vi "Vision Processing.vi"(4 "error in (no error)":errorcluster) -> ()   [LabVIEW 2013]
doc: "This VI runs in parallel to other tasks. It gets images from the camera, processes them for color or shape and use that information to affect robot behavior."
uses:
  <vilib>/Rock Robotics/WPI/Camera/WPI_CameraImageSize.ctl
  Robot Global Data.vi
  <vilib>/vision/NI_Vision_Development_Module.lvlib
panel:
  out "Distance, Angles out":T1(array[cluster])
  in  "Score Limits":T2={"Rect Coverage"=60.0, "X Edge Strength"=40.0, "Y Edge Strength"=60.0, "Center"=75.0, "Outer"=75.0}
  out "Original Image":T3(plugin-control)
  in  "View":bool
  in  "Area Size Limit":i32=444
  in  "Particle Count Limit":i32=10
  in  "Height of target from camera":dbl
  out "Annotated Image":T3(plugin-control)
  in  "Processing":enum32{"Color", "Intensity"}(tab)
  in  "Luminance":i32=200
  in  "Saturation":i32=50
  in  "Hue":i32(knob)=121 scale=0.0..255.0
  in  "Margins":cluster{"Hue":i32, "Sat":i32, "Lum":i32}={"Hue"=40, "Sat"=40, "Lum"=20} {"Sat" scale=0.0..40.0; "Lum" scale=0.0..40.0; "Hue" scale=0.0..40.0}
  # "This is unit-insensitive, outputs in whatever unit you feed it."
  # "Yeah, um, don't use this.\n\n[We never have, so...]"
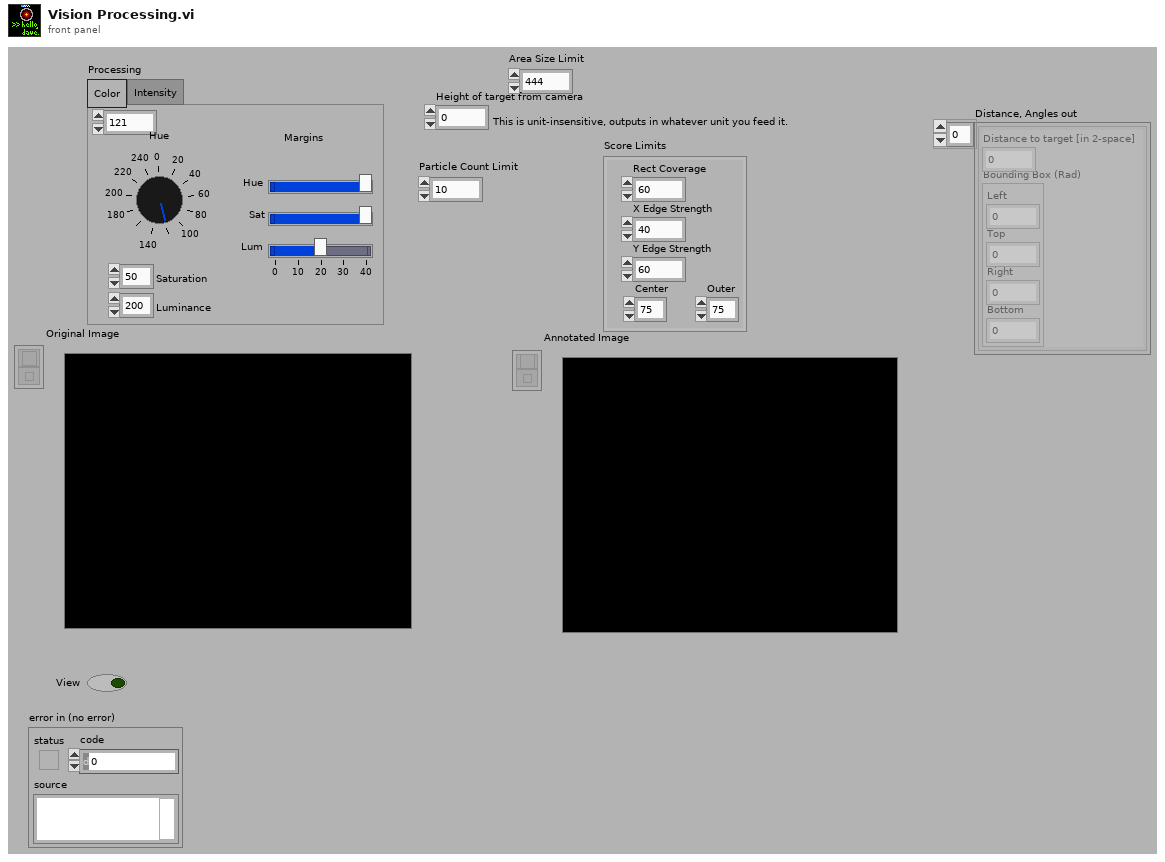
[diagram p1: front panel]
types:
  T1 = cluster{"Distance to target [in 2-space]":dbl, "Bounding Box (Rad)":cluster{"Left":dbl, "Top":dbl, "Right":dbl, "Bottom":dbl}}[]
  T2 = cluster{"Rect Coverage":dbl, "X Edge Strength":dbl, "Y Edge Strength":dbl, "Center":dbl, "Outer":dbl}
  T3 = typedef "IMAQ Image.ctl" = refnum<image>
  T4 = typedef "Image Type" = u32
  T5 = typedef "WPI_CameraDevRef.ctl" = cluster{"Camera Address":string, "CameraStatus":errorcluster, "Acquire Image Notifier":refnum<notifier>}
  T6 = typedef "CameraResolutionInfo.ctl" = cluster{"X Image Resolution":i32, "Y Image Resolution":i32, "FoV X":dbl, "FoV Y":dbl, "X scale":dbl, "Y scale":dbl}
  T7 = typedef "WPI_CameraImageSize.ctl" = enum16{"640x480", "320x240", "160x120"}
  T8 = cluster{cluster{"Left":dbl, "Top":dbl, "Right":dbl, "Bottom":dbl}, "Scores":dbl[], cluster{"Long":dbl, "Short":dbl}}[]
  T9 = cluster{"Left":dbl, "Top":dbl, "Right":dbl, "Bottom":dbl}
  T10 = cluster{"Scores[0]":dbl, "Scores[1]":dbl, "Scores[2]":dbl, "Scores[3]":dbl, "Scores[4]":dbl, "Scores[5]":dbl, "Scores[6]":dbl, "Scores[7]":dbl, "Scores[8]":dbl}
  T11 = cluster{"Distance to target [in 2-space]":dbl, "Bounding Box (Rad)":cluster{"Left":dbl, "Top":dbl, "Right":dbl, "Bottom":dbl}}
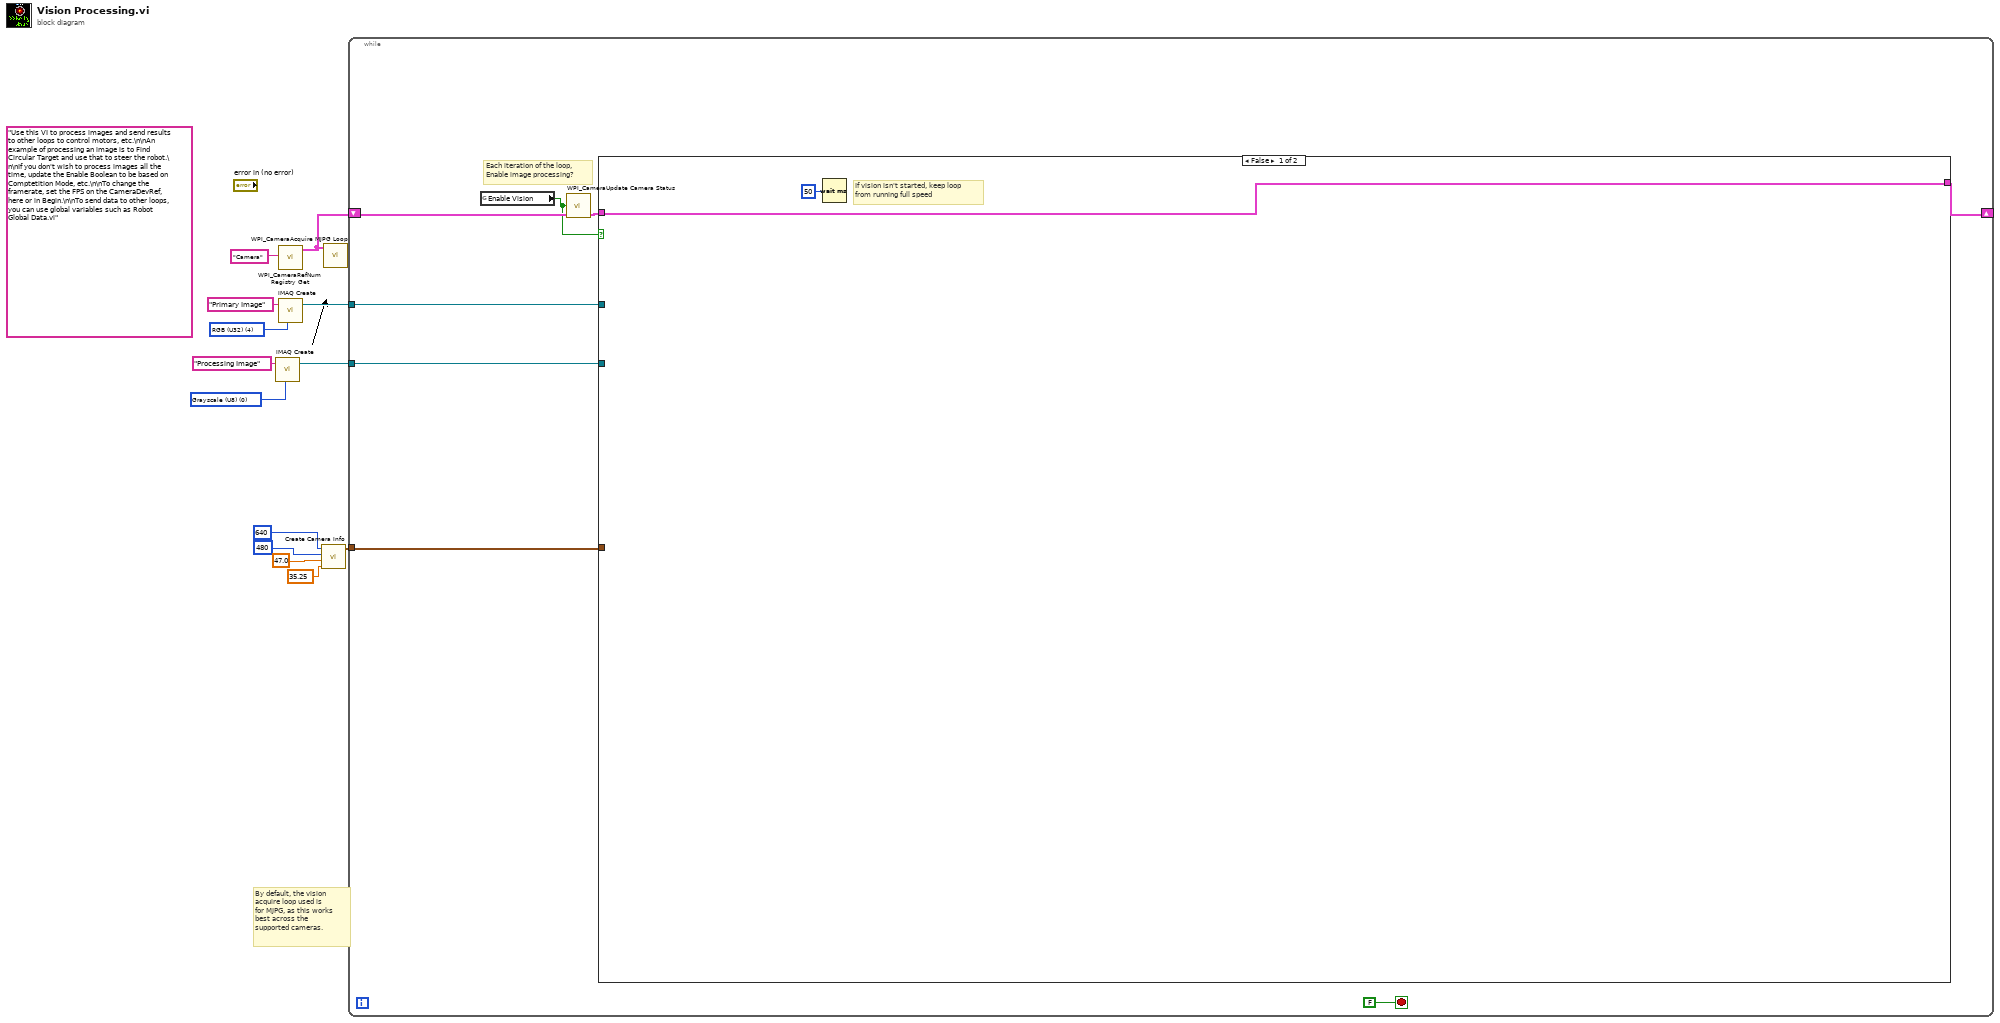
[diagram p0: block diagram]
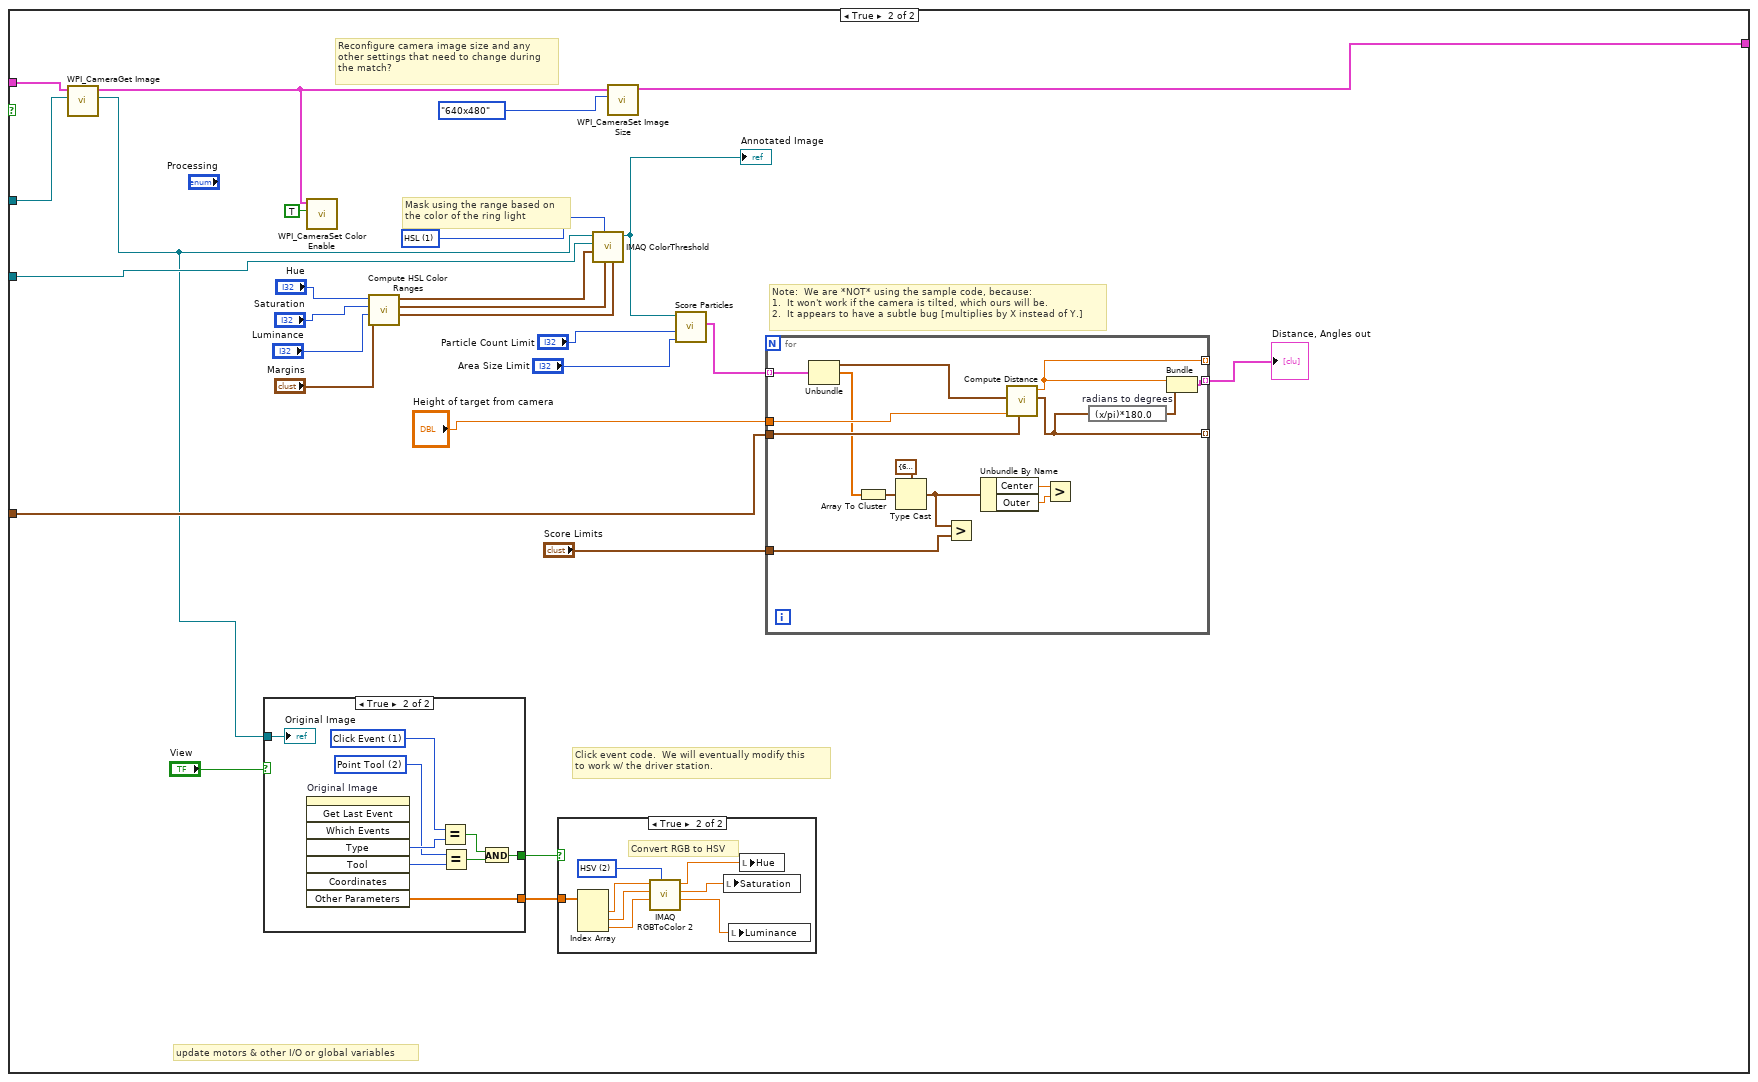
[diagram p2: hidden frame]
diagram:
  w5 = T4 0 items=["Grayscale (U8)", "Grayscale (I16)", "Grayscale (SGL)", "Complex (CSG)", "RGB (U32)", "HSL (U32)", "RGB (U64)"] ("Image Type")
  w7 = T4 4 items=["Grayscale (U8)", "Grayscale (I16)", "Grayscale (SGL)", "Complex (CSG)", "RGB (U32)", "HSL (U32)", "RGB (U64)"] ("Image Type")
  (unwired) "Use this VI to process images and send results to other loops to control motors, etc.\n\nAn example of processing an image is to Find Circular Target and use that to steer the robot.\n\nIf you don't wish to process images all the time, update the Enable Boolean to be based on Comptetition Mode, etc.\n\nTo change the framerate, set the FPS on the CameraDevRef, here or in Begin.\n\nTo send data to other loops, you can use global variables such as Robot Global Data.vi"
  # "By default, the vision\nacquire loop used is\nfor MJPG, as this works\nbest across the\nsupported cameras."
  n1 = call "IMAQ Create"("Image Name"="Processing Image", "Image Type"=w5) -> ("New Image"=w12:T3)  [unwired: 2 in, 2 out]
  n2 = call <vilib>:"WPI_CameraRefNum Registry Get.vi"("refnum name"="Camera") -> ("CameraDevRef"=w8:T5)  [unwired: 1 in, 9 out]
  n3 = call "IMAQ Create"("Image Name"="Primary Image", "Image Type"=w7) -> ("New Image"=w13:T3)  [unwired: 2 in, 2 out]
  n4 = call "Create Camera Info.vi"("FoV Y"=35.25 ("FoV X"), "FoV X"=47.0, "Y Image Resolution"=480, "X Image Resolution"=640) -> ("Camera Info"=w11:T6)  [unwired: 7 in]
  n5 = call <vilib>:"WPI_CameraAcquire MJPG Loop.vi"("CameraDevRef"=w8) -> ()  [unwired: 11 in]
  n6 = while {
    shift-right: [w20] -> _
    shift-left: w8 -> [w18]
    tunnel: w13 -> [w19]
    tunnel: w12 -> [w17]
    tunnel: w11 -> [w16]
    stop <- FALSE stop-if-true
    # "Each iteration of the loop,\nEnable image processing?"
    n7 = global read "Robot Global Data.vi" "Enable Vision"() -> (w14:bool)
    n8 = call <vilib>:"WPI_CameraUpdate Camera Status.vi"("CameraDevRef In"=w18, "Enable Vision"=w14) -> ("CameraDevRef Out"=w15:T5)  [unwired: 3 in]
    n9 = case shown="False" w14 {
      tunnel: w19 -> [_ w49]
      tunnel: [w23 w50] -> w20
      tunnel: w15 -> [w23 w48]
      tunnel: w17 -> [_ w46]
      tunnel: w16 -> [_ w45]
      frame False {
        # "If vision isn't started, keep loop\nfrom running full speed"
        n10 = Wait (ms)(milliseconds to wait=u32 50) -> ()  [unwired: 1 out]
      }
      frame True {
        w39 = u16 1 items=["RGB", "HSL", "HSV", "HSI"] ("Color Mode")
        # "Note:  We are *NOT* using the sample code, because:\n1.  It won't work if the camera is tilted, which ours will be.\n2.  It appears to have a subtle bug [multiplies by X instead of Y.]"
        # "Mask using the range based on\nthe color of the ring light"
        # "Click event code.  We will eventually modify this\nto work w/ the driver station."
        # "update motors & other I/O or global variables"
        # "Reconfigure camera image size and any\nother settings that need to change during\nthe match?"
        n11 = call <vilib>:"WPI_CameraGet Image.vi"("Image"=w49, "CameraDevRef"=w48) -> ("Image Out"=w40:T3, "CameraDevRef Out"=w47:T5)  [unwired: 1 in, 7 out]
        n12 = case shown="True" "View" {
          tunnel: [_ w63] -> w43
          tunnel: [_ w60] -> w42
          tunnel: w40 -> [_ w59]
          frame False {
          }
          frame True {
            w61 = 2 items=["None", "Selection Tool", "Point Tool", "Line Tool", "Rectangle Tool", "Oval Tool", "Polygon Tool", "ClosedFreehandTool", "Annulus Tool", "Rotated Rectangle Tool", "Zoom Tool", "Pan Tool", "Polyline Tool", "Freehand Tool"] ("Tool")
            w62 = 1 items=["No Event"=0, "Click Event"=1, "Draw Event"=2, "Size Event"=4, "Scroll Event"=5, "Double Click Event"=8] ("Type")
            n13 = invoke on="Original Image" class="ImageControl" method="Get Last Event"() -> ("Type"=w64:i32, "Tool"=w67:i32, "Other Parameters"=w60:sgl[])  [unwired: 8 in, 5 out]
            n14 = Equal?(x=w62, y=w64) -> (x = y?=w65:bool)
            n15 = Equal?(x=w61, y=w67) -> (x = y?=w66:bool)
            n16 = And(x=w65, y=w66) -> (x .and. y?=w63:bool)
            "Original Image" <- w59
          }
        }
        n17 = call <vilib>:"WPI_CameraSet Color Enable.vi"("Color Enabled"=TRUE, "CameraDevRef"=w47) -> ()  [unwired: 8 in, 2 out]
        n18 = call "Compute HSL Color Ranges.vi"("Margins"="Margins", "Luminance"="Luminance", "Saturation"="Saturation", "Hue"="Hue") -> ("Lum Range"=w25:cluster{i32, i32}, "Sat Range"=w24:cluster{i32, i32}, "Hue Range"=w26:cluster{i32, i32})  [unwired: 5 in]
        n19 = case shown="True" w43 {
          tunnel: w42 -> [_ w58]
          frame False {
          }
          frame True {
            w57 = u16 2 items=["RGB", "HSL", "HSV", "HSI", "CIE L*a*b*", "CIE XYZ"] ("Color Mode")
            # "Convert RGB to HSV"
            n20 = Index Array(array=w58) -> (element #1=w56:sgl, element #2=w55:sgl, element #3=w54:sgl)  [unwired: 3 in]
            n21 = call "IMAQ RGBToColor 2"("Color Mode"=w57, "Blue value"=w54, "Green value"=w55, "Red value"=w56) -> ("Blue or Luma or Val or Inten or Z or b*value"=w51:dbl, "Green or Sat or Y or a* value"=w52:dbl, "Red or Hue or X or L* value"=w53:dbl)  [unwired: 4 in, 1 out]
            n22 = local write "Saturation"(w52) -> ()
            n23 = local write "Luminance"(w51) -> ()
            n24 = local write "Hue"(w53) -> ()
          }
        }
        n25 = call "IMAQ ColorThreshold"("Blue or Luma or Val or Inten Range"=w25, "Green or Sat Range"=w24, "Color Mode"=w39, "Red or Hue Range"=w26, "Image Dst"=w46, "Image Src"=w40) -> ("Image Dst Out"=w34:T3)  [unwired: 4 in, 1 out]
        "Annotated Image" <- w34
        n26 = call <vilib>:"WPI_CameraSet Image Size.vi"("Image Size"=WPI_CameraImageSize."640x480", "CameraDevRef"=w47) -> ("CameraDevRef Out"=w50:T5)  [unwired: 1 in, 8 out]
        n27 = call "Score Particles.vi"("Area Size Limit"="Area Size Limit", "Particle Count Limit"="Particle Count Limit", "Image Refnum in"=w34) -> ("Scored Particle Info"=w37:T8)  [unwired: 7 in, 1 out]
        n28 = for {
          tunnel: w37 -> [w82] mode=indexing
          tunnel: [w71] -> _ mode=indexing
          tunnel: [w69] -> _ mode=indexing
          tunnel: w45 -> [w79]
          tunnel: "Height of target from camera" -> [w80]
          tunnel: "Score Limits" -> [w73]
          tunnel: [w70] -> w31 mode=indexing
          n29 = Unbundle(w82) -> (w81:T9, "Scores"=w78:dbl[])  [unwired: 1 out]
          n30 = Array To Cluster(array=w78) -> (cluster=w76:T10)
          n31 = Type Cast(type=T2 {"Rect Coverage"=60.0, "X Edge Strength"=40.0, "Y Edge Strength"=60.0, "Center"=75.0, "Outer"=75.0} ("Score Limits"), x=w76) -> (*(type *) &x=w72:T2)
          n32 = Greater?(x=w72, y=w73) -> ()  [unwired: 1 out]
          n33 = Unbundle By Name(w72) -> ("Center"=w75:dbl, "Outer"=w74:dbl)
          n34 = call "Compute Distance.vi"("Camera Info"=w79, "Height from camera of target"=w80, "Bounding Box"=w81) -> ("Bounding Box (Rad)"=w69:T9, "Distance to target [in 2-space]"=w71:dbl)  [unwired: 7 in]
          n35 = Greater?(x=w75, y=w74) -> ()  [unwired: 1 out]
          n36 = expression code="(x/pi)*180.0" "radians to degrees"(w69) -> (w68:T9)
          n37 = Bundle("Distance to target [in 2-space]"=w71, "Bounding Box (Rad)"=w68) -> (w70:T11)  [unwired: 1 in]
        }
        "Distance, Angles out" <- w31
      }
    }
  }
